vi "Update Stats.vi"(11 "Main Controller Actor in":refnum<class "Main Controller Actor.lvclass">) -> (3 "Main Controller Actor out":refnum<class "Main Controller Actor.lvclass">)   [LabVIEW 2021, in "Main Controller Actor.lvclass"]
uses:
  Main Controller Actor.lvclass
  Main Controller Actor.lvclass/Main Controller Actor.ctl
  <vilib>/ptbypt/NI_PtbyPt.lvlib
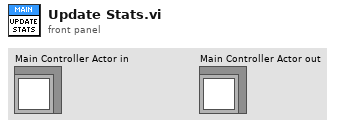
[diagram p1: front panel]
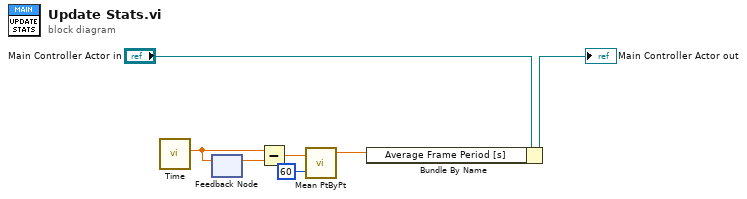
[diagram p0: block diagram]
diagram:
  n1 = call "Time.vi"() -> ("Time [s]"=w1:sgl)  [unwired: 10 in, 1 out]
  n2 = feedback #1() -> (w7:sgl)  [unwired: 1 in]
  n3 = feedback-in #1(w1) -> ()
  n4 = Subtract(x=w1, y=w7) -> (x-y=w4:sgl)
  n5 = call <vilib>:"Mean PtByPt.vi"("x"=w4, "sample length"=60) -> ("mean"=w2:dbl)  [unwired: 2 in, 1 out]
  n6 = Bundle By Name(cluster="Main Controller Actor in", "Average Frame Period [s]"=w2) -> (→"Main Controller Actor out":refnum<class "Main Controller Actor.lvclass">)
